vi "ChooseEstimation.vi"(6 "Time":enum16{"Azul", "Amarelo"}(ring) caption="Enum", 10 "Detection Frame Kalman":T1 {"robots_blue"."height" format="%+4.3f"; "robots_blue"."pixel_y" format="%+4.3f"; "robots_blue"."pixel_x" format="%+4.3f"; "robots_blue"."orientation" format="%+4.3f"; "robots_blue"."y" format="%+4.3f"; "robots_blue"."confidence" format="%4.3f"; "robots_blue"."x" format="%+4.3f"; "robots_yellow"."height" format="%+4.3f"; "robots_yellow"."pixel_y" format="%+4.3f"; "robots_yellow"."pixel_x" format="%+4.3f"; "robots_yellow"."orientation" format="%+4.3f"; "robots_yellow"."y" format="%+4.3f"; "robots_yellow"."confidence" format="%4.3f"; "robots_yellow"."x" format="%+4.3f"}, 11 "Detection Frame Kalman Vel Cmd":T1 {"robots_blue"."height" format="%+4.3f"; "robots_blue"."pixel_y" format="%+4.3f"; "robots_blue"."pixel_x" format="%+4.3f"; "robots_blue"."orientation" format="%+4.3f"; "robots_blue"."y" format="%+4.3f"; "robots_blue"."confidence" format="%4.3f"; "robots_blue"."x" format="%+4.3f"; "robots_yellow"."height" format="%+4.3f"; "robots_yellow"."pixel_y" format="%+4.3f"; "robots_yellow"."pixel_x" format="%+4.3f"; "robots_yellow"."orientation" format="%+4.3f"; "robots_yellow"."y" format="%+4.3f"; "robots_yellow"."confidence" format="%4.3f"; "robots_yellow"."x" format="%+4.3f"}) -> (2 "Detection Frame Out":T1 {"robots_blue"."height" format="%+4.3f"; "robots_blue"."pixel_y" format="%+4.3f"; "robots_blue"."pixel_x" format="%+4.3f"; "robots_blue"."orientation" format="%+4.3f"; "robots_blue"."y" format="%+4.3f"; "robots_blue"."confidence" format="%4.3f"; "robots_blue"."x" format="%+4.3f"; "robots_yellow"."height" format="%+4.3f"; "robots_yellow"."pixel_y" format="%+4.3f"; "robots_yellow"."pixel_x" format="%+4.3f"; "robots_yellow"."orientation" format="%+4.3f"; "robots_yellow"."y" format="%+4.3f"; "robots_yellow"."confidence" format="%4.3f"; "robots_yellow"."x" format="%+4.3f"})   [LabVIEW 2017]
uses:
  SSL Detection Frame.ctl
  SSL Detection Robot.ctl
  <vilib>/Analysis/Matrix/Datatypes/RealMatrix.ctl
  SSL Detection Ball.ctl
  <vilib>/Analysis/_algsub.llb/Real Vector Norm.vi
  <vilib>/ptbypt/NI_PtbyPt.lvlib
  <vilib>/Analysis/NI_AALPro.lvlib
  <vilib>/Analysis/Matrix/NI_Matrix.lvlib
panel:
  out "norm 8":dbl
  out "norm 7":dbl
  out "norm 6":dbl
  out "norm 5":dbl
  out "Waveform Chart":cluster{"norm":dbl}(graph)
  out "norm 4":dbl
  out "norm 3":dbl
  out "norm 2":dbl
  out "norm":dbl
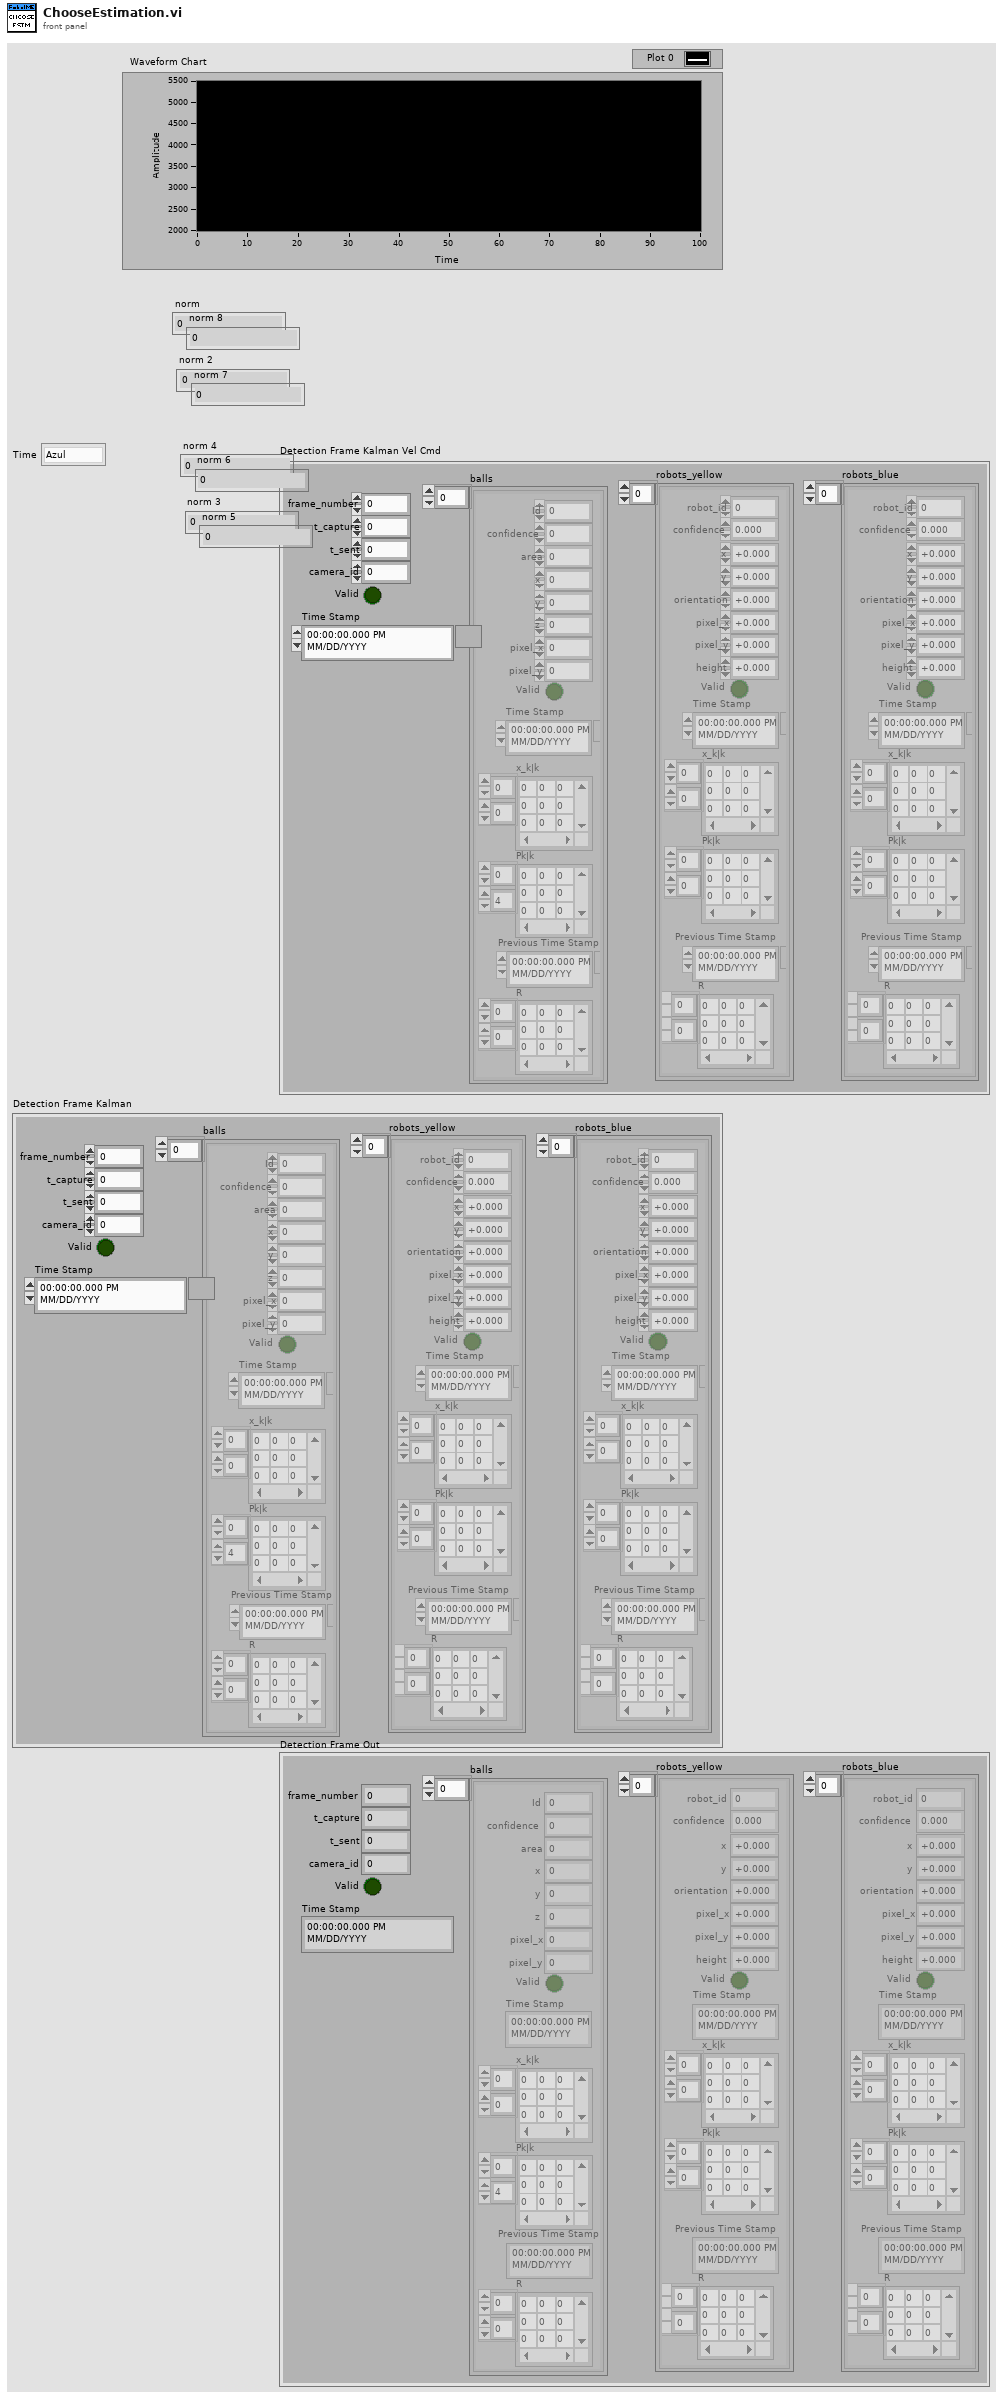
[diagram p1: front panel]
types:
  T1 = typedef "SSL Detection Frame.ctl" = cluster{"frame_number":u32, "t_capture":dbl, "t_sent":dbl, "camera_id":u32, "robots_yellow":T2[], "robots_blue":T2[], "balls":T4[], "Valid":bool, "Time Stamp":timestamp}
  T2 = typedef "SSL Detection Robot.ctl" = cluster{"x":sgl, "robot_id":u32, "confidence":sgl, "y":sgl, "orientation":sgl, "pixel_x":sgl, "pixel_y":sgl, "height":sgl, "Valid":bool, "Time Stamp":timestamp, "x_k|k":T3, "Pk|k":T3, "Previous Time Stamp":timestamp, "R":T3}
  T3 = typedef "NI_Matrix.lvlib/RealMatrix.ctl" = dbl[][]
  T4 = typedef "SSL Detection Ball.ctl" = cluster{"x":sgl, "area":u32, "confidence":sgl, "y":sgl, "z":sgl, "pixel_x":sgl, "pixel_y":sgl, "Valid":bool, "Time Stamp":timestamp, "x_k|k":T3, "Pk|k":T3, "Id":u32, "Previous Time Stamp":timestamp, "R":T3}
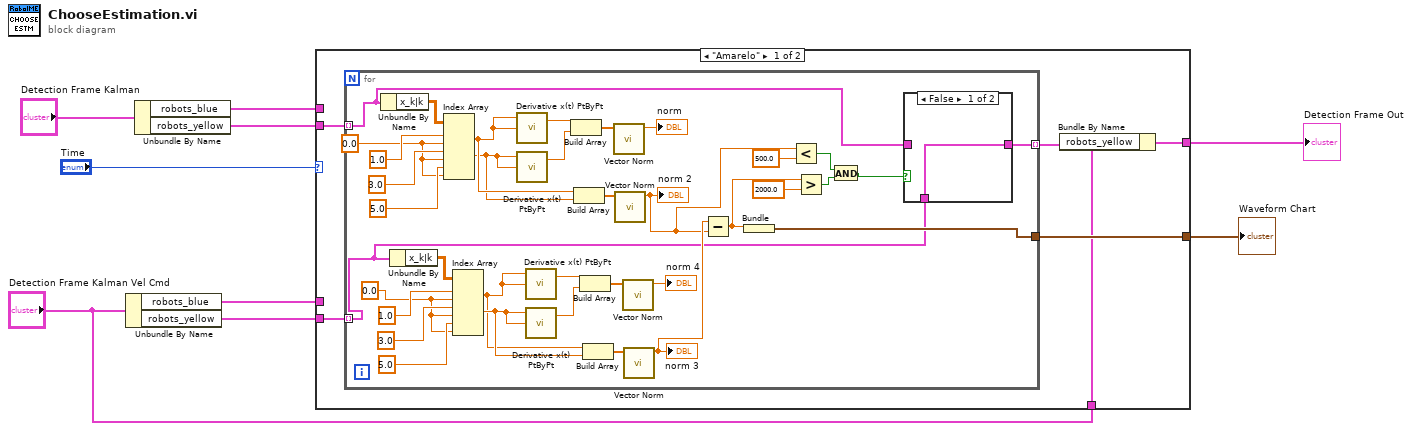
[diagram p0: block diagram]
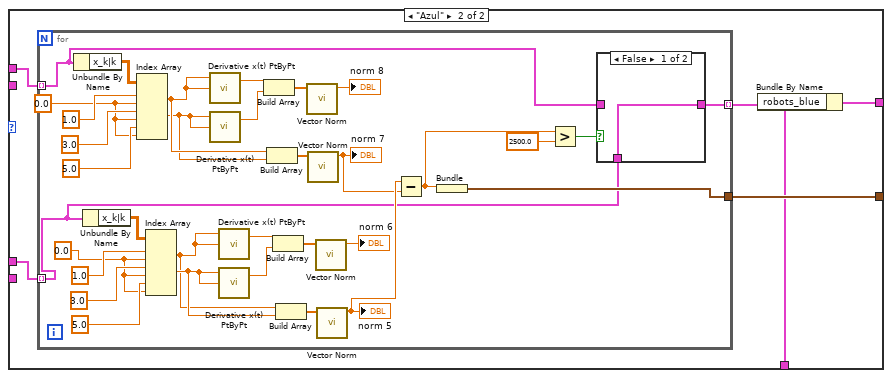
[diagram p3: hidden frame]
diagram:
  n1 = Unbundle By Name("Detection Frame Kalman Vel Cmd") -> ("robots_blue"=w3:T2[], "robots_yellow"=w6:T2[])
  n2 = Unbundle By Name("Detection Frame Kalman") -> ("robots_blue"=w2:T2[], "robots_yellow"=w8:T2[])
  n3 = case shown="\"Amarelo\"" "Time" {
    tunnel: w8 -> [w15 _]
    tunnel: w6 -> [w14 _]
    tunnel: [w13 w59] -> w5
    tunnel: "Detection Frame Kalman Vel Cmd" -> [w12 w58]
    tunnel: [w10 w56] -> w1
    tunnel: w3 -> [_ w55]
    tunnel: w2 -> [_ w54]
    frame "Amarelo" {
      n4 = for {
        tunnel: w15 -> [w23] mode=indexing
        tunnel: w14 -> [w22] mode=indexing
        tunnel: [w28] -> w13
        tunnel: [w21] -> w11 mode=indexing
        w30 = 0.0
        w48 = 0.0
        n5 = Unbundle By Name(w23) -> ("x_k|k"=w47:T3)
        n6 = Unbundle By Name(w22) -> ("x_k|k"=w34:T3)
        n7 = Index Array(array=w47, index (row) #1=1.0, index (col) #1=w48, index (row) #2=3.0, index (col) #2=w48, index (row) #3=5.0, index (col) #3=w48) -> (element #1=w43:dbl, element #2=w42:dbl)  [unwired: 1 out]
        n8 = Index Array(array=w34, index (row) #1=1.0, index (col) #1=w30, index (row) #2=3.0, index (col) #2=w30, index (row) #3=5.0, index (col) #3=w30) -> (element #1=w38:dbl, element #2=w39:dbl)  [unwired: 1 out]
        n9 = call <vilib>:"Derivative x(t) PtByPt.vi"("initial condition"=w43, "x"=w43) -> ("dx/dt"=w46:dbl)  [unwired: 2 in, 1 out]
        n10 = call <vilib>:"Derivative x(t) PtByPt.vi"("initial condition"=w42, "x"=w42) -> ("dx/dt"=w45:dbl)  [unwired: 2 in, 1 out]
        n11 = call <vilib>:"Derivative x(t) PtByPt.vi"("initial condition"=w38, "x"=w38) -> ("dx/dt"=w35:dbl)  [unwired: 2 in, 1 out]
        n12 = call <vilib>:"Derivative x(t) PtByPt.vi"("initial condition"=w39, "x"=w39) -> ("dx/dt"=w36:dbl)  [unwired: 2 in, 1 out]
        n13 = Build Array(w46, w45) -> (w44:dbl[])
        n14 = Build Array(w43, w42) -> (w41:dbl[])
        n15 = Build Array(w35, w36) -> (w37:dbl[])
        n16 = Build Array(w38, w39) -> (w40:dbl[])
        n17 = call-poly <vilib>:"Vector Norm.vi"("Input Vector"=w44) -> ("norm"=→"norm":dbl)  [unwired: 9 in, 1 out]
        n18 = call-poly <vilib>:"Vector Norm.vi"("Input Vector"=w41) -> ("norm"=w20:dbl)  [unwired: 9 in, 1 out]
        "norm 2" <- w20
        n19 = call-poly <vilib>:"Vector Norm.vi"("Input Vector"=w37) -> ("norm"=→"norm 4":dbl)  [unwired: 9 in, 1 out]
        n20 = call-poly <vilib>:"Vector Norm.vi"("Input Vector"=w40) -> ("norm"=w26:dbl)  [unwired: 9 in, 1 out]
        "norm 3" <- w26
        n21 = Subtract(x=w26, y=w20) -> (x-y=w25:dbl)
        n22 = Bundle(w25) -> (w28:cluster{dbl})  [unwired: 1 in]
        n23 = Less?(x=w20, y=500.0) -> (x < y?=w17:bool)
        n24 = Greater?(x=w25, y=2000.0) -> (0:w18:bool)
        n25 = And(x=w17, y=w18) -> (x .and. y?=w16:bool)
        n26 = case shown="False" w16 {
          tunnel: w23 -> [_ w53]
          tunnel: w22 -> [w52 _]
          tunnel: [w52 w53] -> w21
          frame False {
          }
          frame True {
          }
        }
      }
      n27 = Bundle By Name(cluster=w12, "robots_yellow"=w11) -> (w10:T1)
    }
    frame "Azul" {
      n28 = for {
        tunnel: w54 -> [w62] mode=indexing
        tunnel: w55 -> [w61] mode=indexing
        tunnel: [w69] -> w59
        tunnel: [w60] -> w57 mode=indexing
        w71 = 0.0
        w89 = 0.0
        n29 = Unbundle By Name(w62) -> ("x_k|k"=w88:T3)
        n30 = Unbundle By Name(w61) -> ("x_k|k"=w75:T3)
        n31 = Index Array(array=w88, index (row) #1=1.0, index (col) #1=w89, index (row) #2=3.0, index (col) #2=w89, index (row) #3=5.0, index (col) #3=w89) -> (element #1=w84:dbl, element #2=w83:dbl)  [unwired: 1 out]
        n32 = Index Array(array=w75, index (row) #1=1.0, index (col) #1=w71, index (row) #2=3.0, index (col) #2=w71, index (row) #3=5.0, index (col) #3=w71) -> (element #1=w79:dbl, element #2=w80:dbl)  [unwired: 1 out]
        n33 = call <vilib>:"Derivative x(t) PtByPt.vi"("initial condition"=w84, "x"=w84) -> ("dx/dt"=w87:dbl)  [unwired: 2 in, 1 out]
        n34 = call <vilib>:"Derivative x(t) PtByPt.vi"("initial condition"=w83, "x"=w83) -> ("dx/dt"=w86:dbl)  [unwired: 2 in, 1 out]
        n35 = call <vilib>:"Derivative x(t) PtByPt.vi"("initial condition"=w79, "x"=w79) -> ("dx/dt"=w76:dbl)  [unwired: 2 in, 1 out]
        n36 = call <vilib>:"Derivative x(t) PtByPt.vi"("initial condition"=w80, "x"=w80) -> ("dx/dt"=w77:dbl)  [unwired: 2 in, 1 out]
        n37 = Build Array(w87, w86) -> (w85:dbl[])
        n38 = Build Array(w84, w83) -> (w82:dbl[])
        n39 = Build Array(w76, w77) -> (w78:dbl[])
        n40 = Build Array(w79, w80) -> (w81:dbl[])
        n41 = call-poly <vilib>:"Vector Norm.vi"("Input Vector"=w85) -> ("norm"=→"norm 8":dbl)  [unwired: 9 in, 1 out]
        n42 = call-poly <vilib>:"Vector Norm.vi"("Input Vector"=w82) -> ("norm"=w66:dbl)  [unwired: 9 in, 1 out]
        "norm 7" <- w66
        n43 = call-poly <vilib>:"Vector Norm.vi"("Input Vector"=w78) -> ("norm"=→"norm 6":dbl)  [unwired: 9 in, 1 out]
        n44 = call-poly <vilib>:"Vector Norm.vi"("Input Vector"=w81) -> ("norm"=w67:dbl)  [unwired: 9 in, 1 out]
        "norm 5" <- w67
        n45 = Subtract(x=w67, y=w66) -> (x-y=w64:dbl)
        n46 = Bundle(w64) -> (w69:cluster{dbl})  [unwired: 1 in]
        n47 = Greater?(x=w64, y=2500.0) -> (0:w65:bool)
        n48 = case shown="False" w65 {
          tunnel: w62 -> [_ w94]
          tunnel: w61 -> [w93 _]
          tunnel: [w93 w94] -> w60
          frame False {
          }
          frame True {
          }
        }
      }
      n49 = Bundle By Name(cluster=w58, "robots_blue"=w57) -> (w56:T1)
    }
  }
  "Waveform Chart" <- w5
  "Detection Frame Out" <- w1
